vi "GET_PRO_PRODUCT_IDS.vi"(11 "PRODUCT_ID":string) -> (3 "前序工位":string[](array[string]))   [LabVIEW 2020]
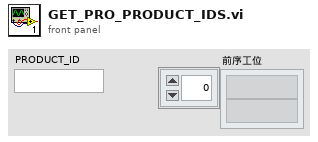
[diagram p1: front panel]
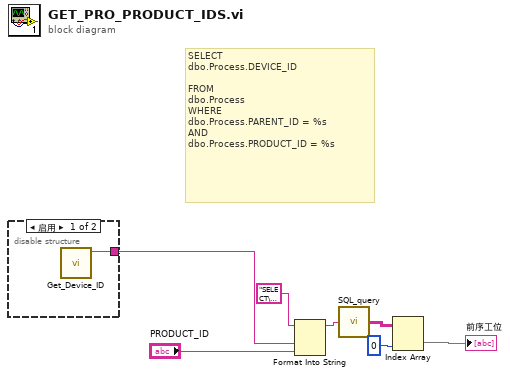
[diagram p0: block diagram]
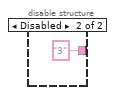
[diagram p2: hidden frame]
diagram:
  # "SELECT\ndbo.Process.DEVICE_ID\n\nFROM\ndbo.Process\nWHERE\ndbo.Process.PARENT_ID = %s\nAND\ndbo.Process.PRODUCT_ID = %s"
  n1 = disable-structure shown="启用" {
    disable-tunnel: [w8 "3" ("Device_ID")] -> w1
    frame Enabled {
      n2 = call "Get_Device_ID.vi"() -> ("Device_ID"=w8:string)  [unwired: 10 in, 1 out]
    }
    frame Disabled {
    }
  }
  n3 = Format Into String(format string="SELECT\ndbo.Process.DEVICE_ID\n\nFROM\ndbo.Process\nWHERE\ndbo.Process.PARENT_ID = %s\nAND\ndbo.Process.PRODUCT_ID = %s" ("SQL query"), w1, "PRODUCT_ID") -> (resulting string=w6:string)  [unwired: 2 in, 1 out]
  n4 = call "SQL_query.vi"("SQL query"=w6) -> ("data"=w5:string[][])  [unwired: 3 in, 1 out]
  n5 = Index Array(array=w5, index (col)=0 ("禁用的索引 (列)")) -> (element=→"前序工位":string[])  [unwired: 1 in]
